vi "SVT UFF58 Read Time Waveform.vi"(0 "function refnum":refnum<k20>, 11 "error in (no error)":errorcluster) -> (3 "ID lines (1-3)":T1, 4 "dup function refnum":refnum<k20>, 6 "waveform":waveform(dbl)(graph), 15 "error out":errorcluster)   [LabVIEW 2017, in "SoundVib_UFF58.lvlib"]
doc: "Reads data from a UFF58 (universal file format) function specified by the <B>function refnum</B> input. This VI also reads the fields in records 1, 2, and 3, returned by ID lines (1-3). You can read a single time domain waveform, a single frequency spectrum, the real and imaginary parts of a frequency spectrum, and any data from a function. The default instance, SVT UFF58 Read Time Waveform, reads a single time domain waveform from a function specified by the <B>function refnum</B> input. Wire data to the <B>function refnum</B> input to determine the polymorphic instance to use or manually select the instance."
uses:
  <vilib>/addons/Sound and Vibration/svt_UFF58/SoundVib_UFF58.lvlib
  <vilib>/addons/Sound and Vibration/svt_UFF58/subVIs/sv_IDLines123.ctl
  <vilib>/addons/_NISVFA/_Shared subVIs/Controls/svc_Channel Info.ctl
  <vilib>/addons/_NISVFA/_Shared subVIs/Controls/svc_Engineering Units Text Ring.ctl
  <vilib>/addons/_NISVFA/_Shared subVIs/Controls/svc_Weighting Filter Text Ring.ctl
  <vilib>/addons/_NISVFA/_Shared subVIs/Common/svc_Set SV Channel Info (variant).vi
  <vilib>/addons/_NISVFA/_Shared subVIs/Common/SVL Set dB Reference (variant).vi
  <vilib>/addons/_NISVFA/_Shared subVIs/Common/svc_Engineering Units to Unit Label.vi
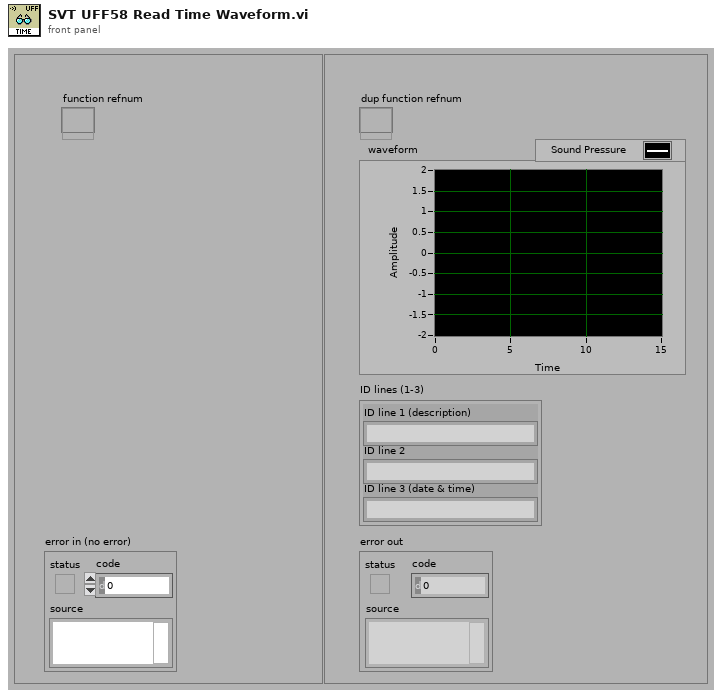
[diagram p1: front panel]
types:
  T1 = typedef "SoundVib_UFF58.lvlib/sv_IDLines123.ctl" = cluster{"ID line 1 (description)":string, "ID line 2":string, "ID line 3 (date & time)":string}
  T2 = typedef "svc_Channel Info.ctl" = cluster{"sensor sensitivity":dbl, "engineering units":T3, "dB reference":dbl, "custom label":string, "weighting filter":T4, "pregain":dbl}
  T3 = typedef "svc_Engineering Units Text Ring.ctl" = u16
  T4 = typedef "svc_Weighting Filter Text Ring.ctl" = u16
  T5 = typedef "SoundVib_UFF58.lvlib/sv_UFF58 DOF.ctl" = cluster{"function type":T6, "function ID number":i32, "version number":i32, "load case ID number":i32, "response entity name":string, "response node":i32, "response direction":T7, "reference entity name":string, "reference node":i32, "reference direction":T7}
  T6 = typedef "SoundVib_UFF58.lvlib/sv_FunctionType.ctl" = enum16{"general or unknown", "time response", "auto spectrum", "cross spectrum", "frequency response function", "transmissibility", "coherence", "auto correlation", "cross correlation", "power spectral density (PSD)", "energy spectral density (ESD)", "probability density function", "spectrum", "cumulative frequency distribution", "peaks valley", "stress/cycles", "strain/cycles", "orbit", "mode indicator function", "force pattern", "partial power", "partial coherence", "eigenvalue", "eigenvector", "shock response spectrum", "finite impulse response filter", "multiple coherence", "order function", "phase compensation"}
  T7 = typedef "SoundVib_UFF58.lvlib/sv_UFF58 Response Direction.ctl" = i32
  T8 = typedef "SoundVib_UFF58.lvlib/sv_UFF58 Data Form.ctl" = cluster{"ordinate data type":u16, "number of data values/pairs":i32, "abscissa spacing":enum16{"uneven", "even"}, "abscissa minimum":dbl, "abscissa increment":dbl}
  T9 = typedef "SoundVib_UFF58.lvlib/sv_UFF58 Axis Characteristics.ctl" = cluster{"specific data type":T10, "length units exponent":i32, "force units exponent":i32, "temperature units exponent":i32, "axis label":string, "axis units label":string}
  T10 = typedef "SoundVib_UFF58.lvlib/sv_UFF58 Specific Datatype.ctl" = u16
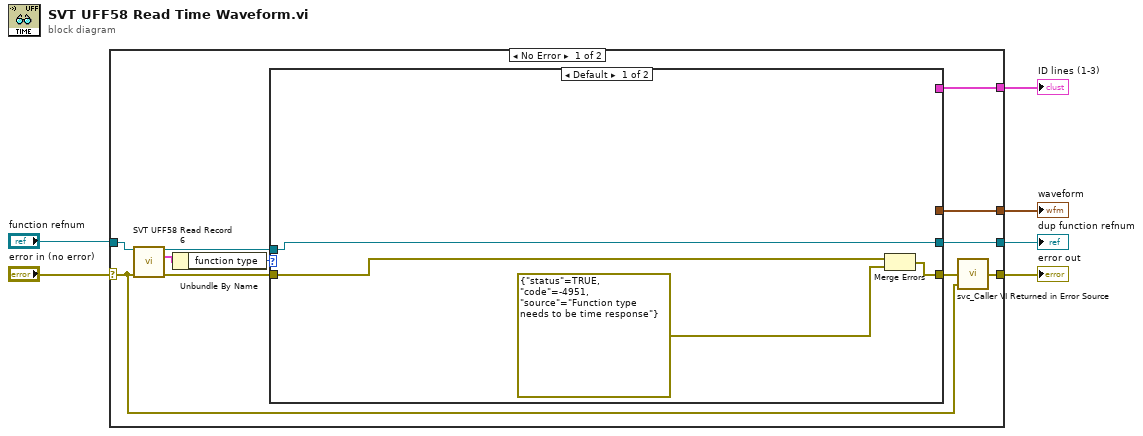
[diagram p0: block diagram]
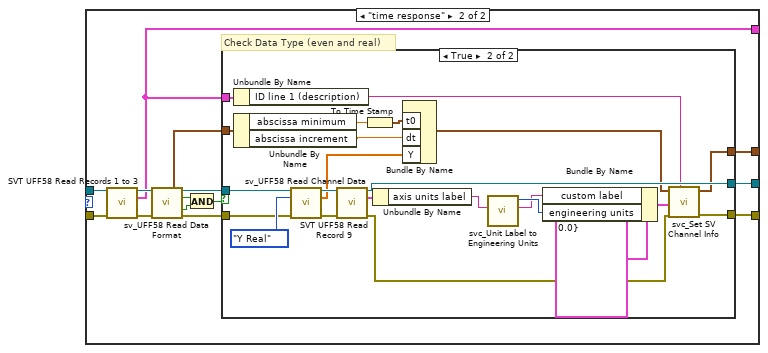
[diagram p2: hidden frame]
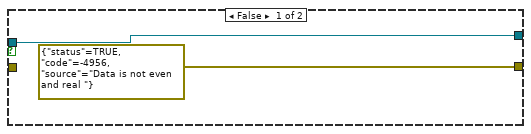
[diagram p3: hidden frame]
diagram:
  n1 = case shown="No Error" "error in (no error)" {
    selector: "error in (no error)" -> [w8 w62]
    tunnel: [w17 w61] -> w1
    tunnel: [w9 w62] -> w6
    tunnel: "function refnum" -> [w13 w61]
    tunnel: [w16 _] -> w4
    tunnel: [w7 _] -> w3
    frame No Error {
      n2 = call <vilib>:"SVT UFF58 Read Record 6.vi"("function refnum"=w13, "error in (no error)"=w8) -> ("dup function refnum"=w12:refnum<k20>, "DOF identification"=w15:T5, "error out"=w14:errorcluster)  [unwired: 11 in]
      n3 = Unbundle By Name(w15) -> ("function type"=w11:T6)
      n4 = case shown="Default" w11 {
        tunnel: [w21 w26] -> w17
        tunnel: [w18 w25] -> w10
        tunnel: [_ w23] -> w16
        tunnel: w14 -> [w20 w31]
        tunnel: w12 -> [w21 w30]
        tunnel: [_ w22] -> w7
        frame Default {
          n5 = Merge Errors(w20, errorcluster {"status"=TRUE, "code"=-4951, "source"="Function type needs to be time response"} ("error out")) -> (w18:errorcluster)
        }
        frame "time response" {
          # "Check Data Type (even and real)"
          n6 = call <vilib>:"SVT UFF58 Read Records 1 to 3.vi"("function refnum"=w30, "error in (no error)"=w31) -> ("dup function refnum"=w33:refnum<k20>, "ID lines (1-3)"=w23:T1, "error out"=w32:errorcluster)  [unwired: 11 in]
          n7 = call <vilib>:"sv_UFF58 Read Data Format.vi"("function refnum"=w33, "error in (no error)"=w32) -> ("data form"=w24:T8, "dup function refnum"=w35:refnum<k20>, "even"=w28:bool, "real"=w29:bool, "error out"=w34:errorcluster)  [unwired: 9 in]
          n8 = And(x=w28, y=w29) -> (x .and. y?=w27:bool)
          n9 = case shown="True" w27 {
            tunnel: w35 -> [w37 w55]
            tunnel: w34 -> [_ w54]
            tunnel: [w37 w60] -> w26
            tunnel: [errorcluster {"status"=TRUE, "code"=-4956, "source"="Data is not even and real "} ("error out") w49] -> w25
            tunnel: w24 -> [_ w53]
            tunnel: w23 -> [_ w50]
            tunnel: [_ w47] -> w22
            frame False {
            }
            frame True {
              n10 = Unbundle By Name(w50) -> ("ID line 1 (description)"=w46:string)
              n11 = Unbundle By Name(w53) -> ("abscissa minimum"=w52:dbl, "abscissa increment"=w51:dbl)
              n12 = call <vilib>:"sv_UFF58 Read Channel Data.vi"("function refnum"=w55, "channel to read"=enum16{"X", "Y Real", "Y Imaginary"}."Y Real" ("data to read"), "error in (no error)"=w54) -> ("dup function refnum"=w59:refnum<k20>, "data"=w58:dbl[], "error out"=w45:errorcluster)  [unwired: 10 in]
              n13 = call <vilib>:"SVT UFF58 Read Record 9.vi"("function refnum"=w59, "error in (no error)"=w45) -> ("dup function refnum"=w60:refnum<k20>, "ordinate data characteristics"=w44:T9, "error out"=w41:errorcluster)  [unwired: 11 in]
              n14 = To Time Stamp(1:w52) -> (0:w57:timestamp)
              n15 = Unbundle By Name(w44) -> ("axis units label"=w40:string)
              n16 = Bundle By Name("t0"=w57, "dt"=w51, "Y"=w58) -> (w48:waveform(dbl))  [unwired: 1 in]
              n17 = call <vilib>:"svc_Unit Label to Engineering Units.vi"("unit label"=w40) -> ("unit label out"=w38:string, "engineering units"=w39:T3)  [unwired: 9 in]
              n18 = Bundle By Name(cluster=T2 {"sensor sensitivity"=1000.0, "engineering units"=0, "dB reference"=1.0, "custom label"="EU", "weighting filter"=0, "pregain"=0.0} ("channel info"), "custom label"=w38, "engineering units"=w39) -> (w42:T2)
              n19 = call <vilib>:"svc_Set SV Channel Info.vi"("channel name"=w46, "error in (no error)"=w41, "channel info"=w42, "scaled signal in"=w48) -> ("error out"=w49:errorcluster, "scaled signal out"=w47:waveform(dbl))  [unwired: 6 in]
            }
          }
        }
      }
      n20 = call <vilib>:"svc_Caller VI Returned in Error Source.vi"("warning input to caller"=w8, "error in (no error)"=w10) -> ("error out"=w9:errorcluster)  [unwired: 3 in]
    }
    frame Error {
    }
  }
  "error out" <- w6
  "waveform" <- w3
  "ID lines (1-3)" <- w4
  "dup function refnum" <- w1
